vi "TrfcLit.vi"(9 "Interval 2":u32=500, 10 "Reset/Red? 2":bool=TRUE, 11 "ColorBox in":refnum<vi>) -> ()   [LabVIEW 2024]
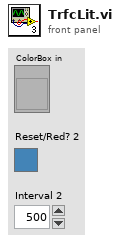
[diagram p1: front panel]
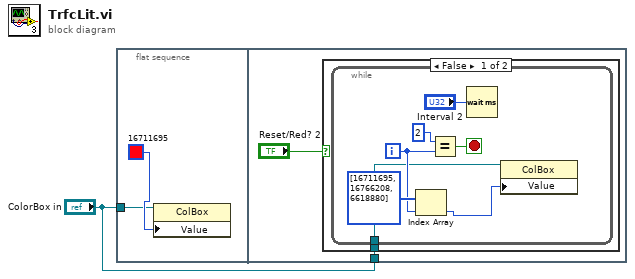
[diagram p0: block diagram]
diagram:
  n1 = flat-sequence {
    tunnel: "ColorBox in" -> [w2]
    tunnel: "ColorBox in" -> [w4]
    frame #0 {
      n2 = property class="ColBox"(reference=w2, "Value"=u32 16711695 ("Color Box")) -> ()  [unwired: 1 in, 2 out]
    }
    frame #1 {
      n3 = case shown="False" "Reset/Red? 2" {
        tunnel: w4 -> [w6 _]
        frame False {
          n4 = while {
            tunnel: w6 -> [w7]
            i -> [w11]
            stop <- w9 stop-if-true
            n5 = Index Array(array=u32[] [16711695, 16766208, 6618880] ("Array 2"), index=w11) -> (element=w8:u32)
            n6 = Equal?(x=2, y=w11) -> (x = y?=w9:bool)
            n7 = Wait (ms)(milliseconds to wait="Interval 2") -> ()  [unwired: 1 out]
            n8 = property class="ColBox"(reference=w7, "Value"=w8) -> ()  [unwired: 1 in, 2 out]
          }
        }
        frame True {
        }
      }
    }
  }
